vi "Output 信息提取.vi"(10 "输出":T1) -> (2 "Output 信息配置":string[](array[string]))   [LabVIEW 2017]
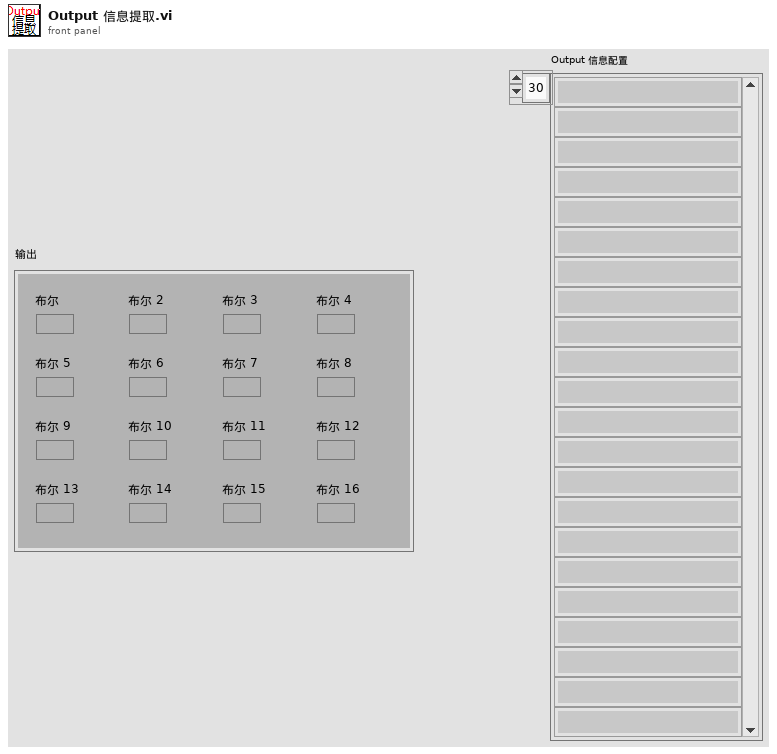
[diagram p1: front panel]
types:
  T1 = typedef "output控件.ctl" = cluster{"布尔":bool, "布尔 2":bool, "布尔 3":bool, "布尔 4":bool, "布尔 5":bool, "布尔 6":bool, "布尔 7":bool, "布尔 8":bool, "布尔 9":bool, "布尔 10":bool, "布尔 11":bool, "布尔 12":bool, "布尔 13":bool, "布尔 14":bool, "布尔 15":bool, "布尔 16":bool}
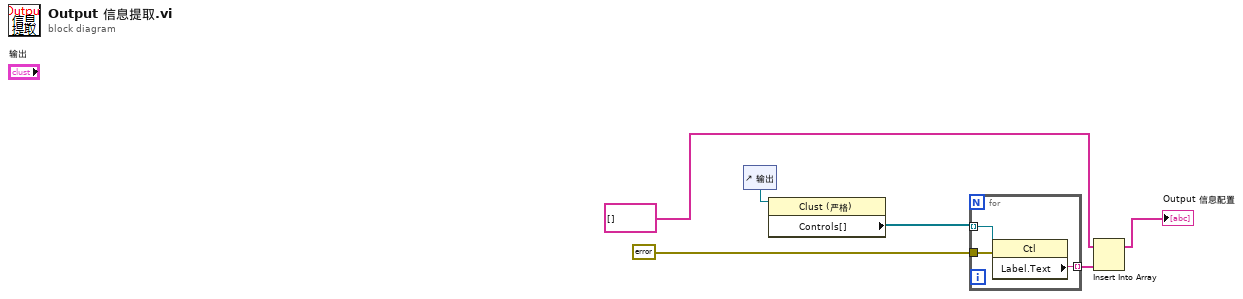
[diagram p0: block diagram]
diagram:
  n1 = control-ref of="输出"() -> (w1:refnum<vi>)
  n2 = property class="Clust (严格)"(reference=w1) -> ("Controls[]"=w3:refnum<vi>[])  [unwired: 1 in, 2 out]
  n3 = for {
    tunnel: w3 -> [w9] mode=indexing
    tunnel: errorcluster {"status"=FALSE, "code"=0, "source"=""} ("错误输入（无错误）") -> [w8]
    tunnel: [w7] -> w2 mode=indexing
    n4 = property class="Ctl"(reference=w9, error in=w8) -> ("Label.Text"=w7:string)  [unwired: 2 out]
  }
  n5 = Insert Into Array(array=string[] [], new element=w2) -> (→"Output 信息配置":string[])  [unwired: 1 in]
